vi "etc_XCITE_SetLogFile.vi"(8 "error in (no error)":errorcluster {"code" format="%x"}, 11 "name":string) -> (0 "error out":errorcluster {"code" format="%x"})   [LabVIEW 2019, in "XCite.lvlib"]
doc: "Sends a command to execute on the slelected X-cite device."
uses:
  XCite.lvlib
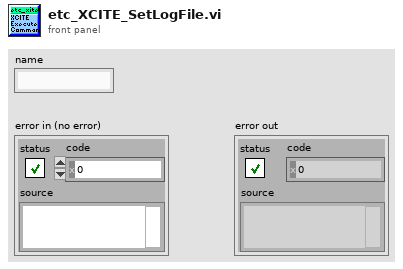
[diagram p1: front panel]
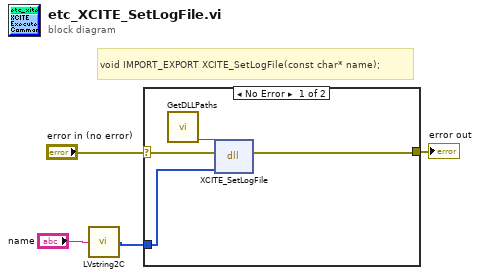
[diagram p0: block diagram]
diagram:
  # "void IMPORT_EXPORT XCITE_SetLogFile(const char* name);"
  n1 = call "LVstring2C.vi"("LVString"="name") -> ("CString"=w1:u8[])  [unwired: 3 in, 1 out]
  n2 = case shown="No Error" "error in (no error)" {
    selector: "error in (no error)" -> [w8 w9]
    tunnel: [w5 w9] -> w4
    tunnel: w1 -> [w6 _]
    frame No Error {
      n3 = call "GetDLLPaths.vi"() -> ("etc_xcite_path"=w7:path)  [unwired: 8 in, 3 out]
      n4 = dll-call lib="C:/LabVIEWDevFall2024/pco.labview/labview_sdk/runtime/bin64/etc_xcite.dll" fn="XCITE_SetLogFile"(path in=w7, error in=w8, "name"=w6) -> (error out=w5:errorcluster)  [unwired: 3 in, 1 out]
    }
    frame Error {
    }
  }
  "error out" <- w4
